vi "AllocateImageBuffer.vi"(0 "Camera Session":T3, 1 "Required num frames":u32=100, 2 "Camera Control":T1={"Acquisition Freq"=30.0, "Exposure (ms)"=10.0, "Gain"=10.0, "Height"=1200, "Width"=2000, "Acq. trigger start"=TRUE} {"Acquisition Freq" min=1e-06 max=1000.0; "Height" min=400 max=2064 step=1; "Width" min=400 max=3088 step=1}) -> (3 "All Image Buffers":T2[](array[typedef]), 4 "#Frames Buffer":u32=4000, 5 "RAM Needed (GB)":dbl, 6 "Recording Time (s)":dbl)   [LabVIEW 2021]
uses:
  <vilib>/userdefined/High Color/IMAQdx.ctl
  <vilib>/vision/Image Controls.llb/IMAQ Image.ctl
  <vilib>/vision/driver/IMAQdx.llb/IMAQdx Acquisition Mode.ctl
  <vilib>/vision/driver/NI_Vision_Acquisition_Software.lvlib
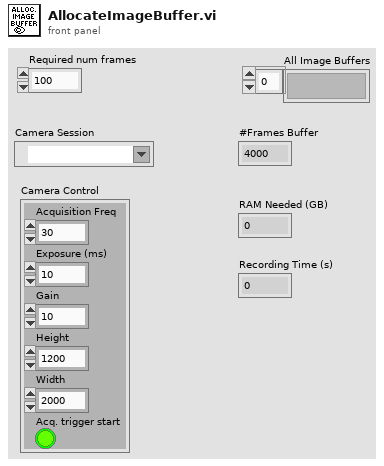
[diagram p1: front panel]
types:
  T1 = cluster{"Acquisition Freq":dbl, "Exposure (ms)":dbl, "Gain":sgl, "Height":u16, "Width":u16, "Acq. trigger start":bool}
  T2 = typedef "IMAQ Image.ctl" = refnum<image>
  T3 = typedef "IMAQdx.ctl" = refnum<k21>
  T4 = typedef "NI_Vision_Acquisition_Software.lvlib/IMAQdx Acquisition Mode.ctl" = enum32{"One Shot", "Continuous"}
  T5 = typedef "Image Type" = u32
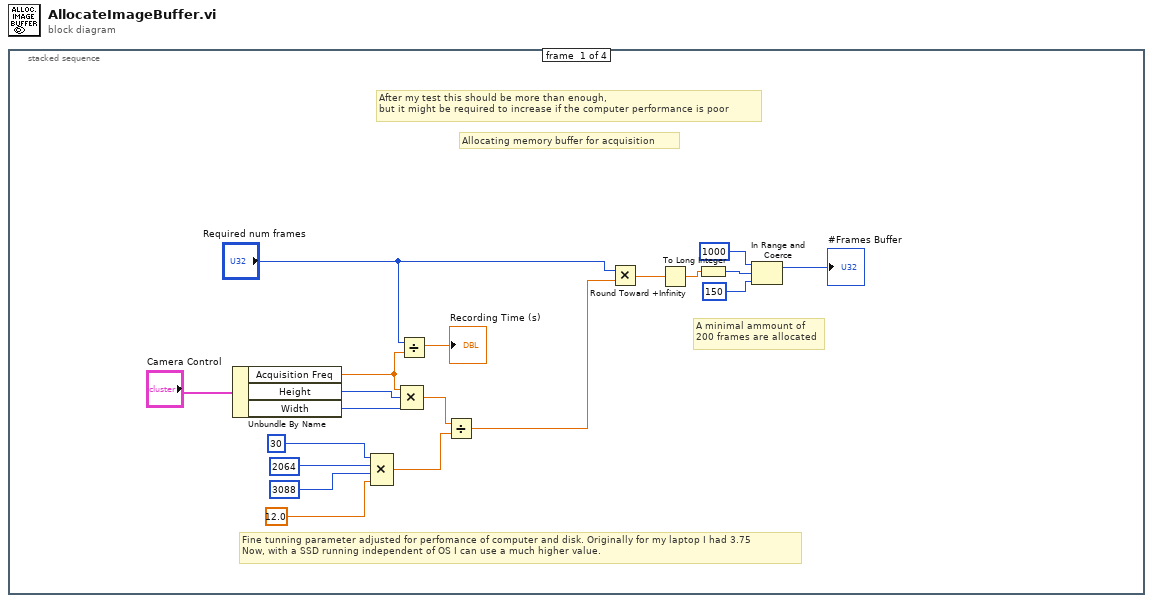
[diagram p0: block diagram]
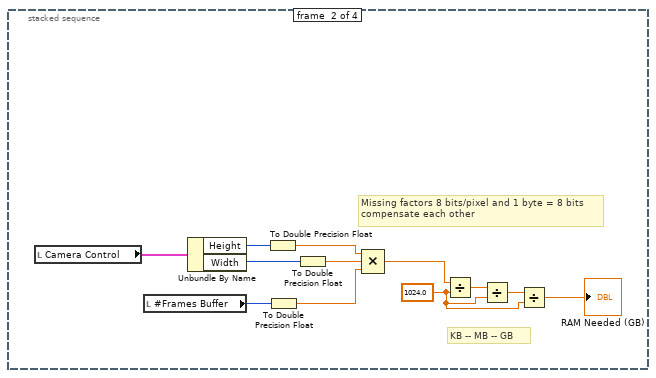
[diagram p2: hidden frame]
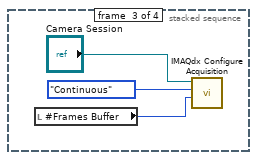
[diagram p3: hidden frame]
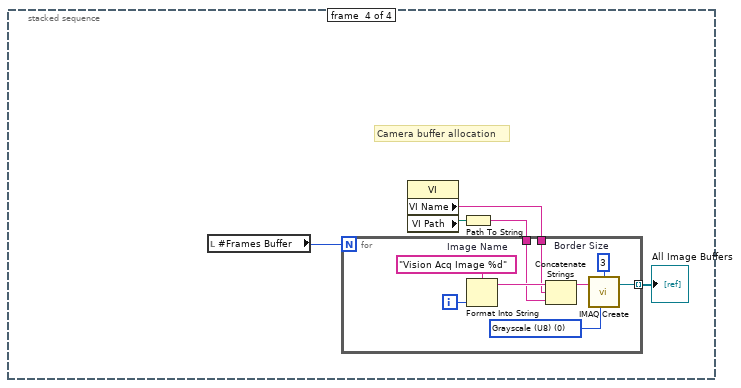
[diagram p4: hidden frame]
diagram:
  n1 = stacked-sequence {
    frame #0 {
      # "Fine tunning parameter adjusted for perfomance of computer and disk. Originally for my laptop I had 3.75\nNow, with a SSD running independent of OS I can use a much higher value."
      # "A minimal ammount of\n200 frames are allocated"
      # "After my test this should be more than enough,\nbut it might be required to increase if the computer performance is poor"
      # "Allocating memory buffer for acquisition"
      n2 = Unbundle By Name("Camera Control") -> ("Acquisition Freq"=w8:dbl, "Height"=w17:u16, "Width"=w16:u16)
      n3 = Compound Arithmetic op=MULTIPLY(30, 2064, 3088, 12.0 ("value")) -> (w11:dbl)
      n4 = Divide(x="Required num frames", y=w8) -> (x/y=→"Recording Time (s)":dbl)
      n5 = Compound Arithmetic op=MULTIPLY(w8, w17, w16) -> (w10:dbl)
      n6 = Divide(x=w10, y=w11) -> (x/y=w12:dbl)
      n7 = Multiply(x="Required num frames", y=w12) -> (x*y=w19:dbl)
      n8 = Round Toward +Infinity(x=w19) -> (ceil(x): smallest int >= x=w4:dbl)
      n9 = To Long Integer(number=w4) -> (32bit integer=w1:i32)
      n10 = In Range and Coerce(upper limit=u32 1000 ("#Frames Buffer"), x=w1, lower limit=150 ("y")) -> (coerced(x)=→"#Frames Buffer":u32)  [unwired: 1 out]
    }
    frame #1 {
      w24 = 1024.0 ("y")
      # "Missing factors 8 bits/pixel and 1 byte = 8 bits\ncompensate each other"
      # "KB -- MB -- GB"
      n11 = local read "Camera Control"() -> (w30:T1)
      n12 = local read "#Frames Buffer"() -> (w27:u32)
      n13 = Unbundle By Name(w30) -> ("Height"=w29:u16, "Width"=w28:u16)
      n14 = To Double Precision Float(number=w29) -> (double precision float=w22:dbl)
      n15 = To Double Precision Float(number=w27) -> (double precision float=w20:dbl)
      n16 = To Double Precision Float(number=w28) -> (double precision float=w21:dbl)
      n17 = Compound Arithmetic op=MULTIPLY(w22, w21, w20) -> (w26:dbl)
      n18 = Divide(x=w26, y=w24) -> (x/y=w31:dbl)
      n19 = Divide(x=w31, y=w24) -> (x/y=w25:dbl)
      n20 = Divide(x=w25, y=w24) -> (x/y=→"RAM Needed (GB)":dbl)
    }
    frame #2 {
      n21 = local read "#Frames Buffer"() -> (w33:u32)
      n22 = call <vilib>:"IMAQdx Configure Acquisition.vi"("Number of Buffers"=w33, "Continuous?"=IMAQdx_Acquisition_Mode."Continuous", "Session In"="Camera Session") -> ()  [unwired: 1 in, 8 out]
    }
    frame #3 {
      # "Camera buffer allocation"
      n23 = local read "#Frames Buffer"() -> (w35:u32)
      n24 = property class="VI"() -> ("VI Name"=w38:string, "VI Path"=w39:path)  [unwired: 2 in, 2 out]
      n25 = Path To String(path=w39) -> (string=w37:string)
      n26 = for "For Loop_template0" {
        N: w35 -> [_]
        tunnel: [w48] -> w36 mode=indexing
        tunnel: w38 -> [w43]
        tunnel: w37 -> [w42]
        i -> [w47]
        w40 = T5 0 items=["Grayscale (U8)", "Grayscale (I16)", "Grayscale (SGL)", "Complex (CSG)", "RGB (U32)", "HSL (U32)", "RGB (U64)", "Grayscale (U16)"] ("Image Type")
        w41 = 3  # Border Size
        w46 = "Vision Acq Image %d"  # Image Name
        n27 = Format Into String(format string=w46, w47) -> (resulting string=w45:string)  [unwired: 2 in, 1 out]
        n28 = Concatenate Strings(w45, w43, w42) -> (w44:string)
        n29 = call "IMAQ Create"("Border Size"=w41, "Image Name"=w44, "Image Type"=w40) -> ("New Image"=w48:T2)  [unwired: 1 in, 2 out]
      }
      "All Image Buffers" <- w36
    }
  }
